vi "Test.vi"() -> ()   [LabVIEW 2014]
doc: "This VI is called when test mode begins, and will automatically be terminated when it ends. You can add manual or automatic tests and invoke them from the dashboard."
uses:
  SensorTestData.ctl
  <vilib>/Rock Robotics/WPI/Ultrasonic/WPI_SonarMB1010DigitalRefNum Registry Get.vi
  <vilib>/Rock Robotics/WPI/Ultrasonic/WPI_SonarMB1010DigitalGetRange.vi
  GyroGlobal.vi
  Elevator System/Public/Sensors Global.vi
  <vilib>/Rock Robotics/Network Tables/SD Write String.vi
  <vilib>/Rock Robotics/WPI/Joystick/WPI_JoystickGetSetRefNum.vi
  <vilib>/Rock Robotics/Network Tables/SD Write Number.vi
  <vilib>/Rock Robotics/WPI/RobotDrive/WPI_RobotDriveGetSetRefNum.vi
  <vilib>/Rock Robotics/Network Tables/SD Write Numeric Array.vi
panel:
  in  "Gripper Power":dbl=0.5 format="%#_13g"
  in  "Elevator Power":dbl=0.5 format="%#_13g"
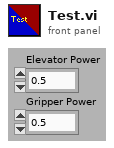
[diagram p1: front panel]
types:
  T1 = typedef "SensorTestData.ctl" = cluster{"EncoderR":dbl, "EncoderL":dbl, "EncoderS":dbl, "Tote Position":bool, "UltrasonicLR":dbl, "UltrasonicHR":dbl, "Gyro Angle":dbl, "Elevator Sensor":dbl, "Gripper Sensor L":dbl, "Gripper Sensor R":dbl}
  T2 = typedef "WPI_PotentiometerDevRef.ctl" = cluster{"DevStatus":errorcluster, "Controller":T3, "Analog Channel":T4, "Invert Output":bool}
  T3 = typedef "FPGA_TypedefAnalogModule.ctl" = enum16{"Controller 1"}
  T4 = typedef "FPGA_AIChannel.ctl" = enum8{"AI 0", "AI 1", "AI 2", "AI 3", "AI MXP 0", "AI MXP 1", "AI MXP 2", "AI MXP 3", "Invalid"}
  T5 = typedef "WPI_EncoderDevRef.ctl" = cluster{"DevStatus":errorcluster, "EncoderIndex":T6, "CounterIndex":T7, "DistancePerCount":dbl, "Decoding Type":T8}
  T6 = typedef "FPGA_EncoderIdx.ctl" = enum8{"Enc 0", "Enc 1", "Enc 2", "Enc 3", "Enc 4", "Enc 5", "Enc 6", "Enc 7", "Invalid"}
  T7 = typedef "FPGA_CounterCtrSystemIndex.ctl" = enum8{"Ctr 0", "Ctr 1", "Ctr 2", "Ctr 3", "Ctr 4", "Ctr 5", "Ctr 6", "Ctr 7", "Invalid"}
  T8 = typedef "WPI_EncoderType.ctl" = enum16{"1x", "2x", "4x"}
  T9 = typedef "WPI_SwitchDevRef.ctl" = cluster{"DevStatus":errorcluster, "DIO Channel":T10, "Controller":T11, "CntIndex":T7, "Normally Closed":bool}
  T10 = typedef "FPGA_DIOChannel.ctl" = enum8{"DIO 0", "DIO 1", "DIO 2", "DIO 3", "DIO 4", "DIO 5", "DIO 6", "DIO 7", "DIO 8", "DIO 9", "DIO MXP 0", "DIO MXP 1", "DIO MXP 2", "DIO MXP 3", "DIO MXP 4", "DIO MXP 5", "DIO MXP 6", "DIO MXP 7", "DIO MXP 8", "DIO MXP 9", "DIO MXP 10", "DIO MXP 11", "DIO MXP 12", "DIO MXP 13", "DIO MXP 14", "DIO MXP 15", "Invalid"}
  T11 = typedef "FPGA_TypedefDigitalModule.ctl" = enum16{"Controller 1"}
  T12 = typedef "WPI_SonarMB1010DigitalDeviceRef.ctl" = cluster{"CounterDevRef":T13, "Scaling factor (s/in)":dbl}
  T13 = typedef "WPI_CounterDevRef.ctl" = cluster{"DevStatus":errorcluster, "CntIndex":T7}
  T14 = typedef "WPI_JoystickDevRef.ctl" = cluster{"Device":T15}
  T15 = typedef "WPI_JoystickDeviceEnum.ctl" = enum16{"USB 0", "USB 1", "USB 2", "USB 3", "USB 4", "USB 5"}
  T16 = typedef "WPI_RobotDriveDevRef.ctl" = cluster{"DevStatus":errorcluster, "Motors[]":T17[], "Square Inputs":bool, "Max Output":dbl}
  T17 = typedef "WPI_MotorControlDeviceRef.ctl" = cluster{"DeviceStatus":errorcluster, "Type":T18, "PWM":cluster{"Controller":T11, "PWM Channel":T19, "DeadBand":T20}, "CAN":cluster{"Device Number":u8, "Control Mode":T21, "Semaphore":T22, "Max Vout":dbl, "TalonSRX Control Mode":T23}, "Invert":bool, "TransformRef":T24, "InvTransformRef":T24}
  T18 = typedef "WPI_MotorControlType.ctl" = enum16{"PWM", "CAN", "CANTalonSRX"}
  T19 = typedef "FPGA_DIOPWMChannel.ctl" = enum8{"PWM 0", "PWM 1", "PWM 2", "PWM 3", "PWM 4", "PWM 5", "PWM 6", "PWM 7", "PWM 8", "PWM 9", "PWM MXP 0", "PWM MXP 1", "PWM MXP 2", "PWM MXP 3", "PWM MXP 4", "PWM MXP 5", "PWM MXP 6", "PWM MXP 7", "PWM MXP 8", "PWM MXP 9", "Invalid"}
  T20 = typedef "WPI_PWMDeadband.ctl" = cluster{"Name":string, "maxPositivePwm":i32, "minPositivePwm":i32, "centerPwm":i32, "maxNegativePwm":i32, "minNegativePwm":i32, "angularRange":u16}
  T21 = typedef "WPI_CANJaguar_ControlMode.ctl" = enum8{"Percent VBus", "Current", "Speed", "Position", "Voltage"}
  T22 = typedef "Semaphore RefNum" = refnum<k1>
  T23 = typedef "WPI_CANTalonSRX_APIControlMode.ctl" = enum8{"Percent VBus", "Speed", "Position", "Slave", "Unchanged / Invalid"}
  T24 = typedef "WPI_PWMTransform_ConPane.ctl" = refnum<vi>
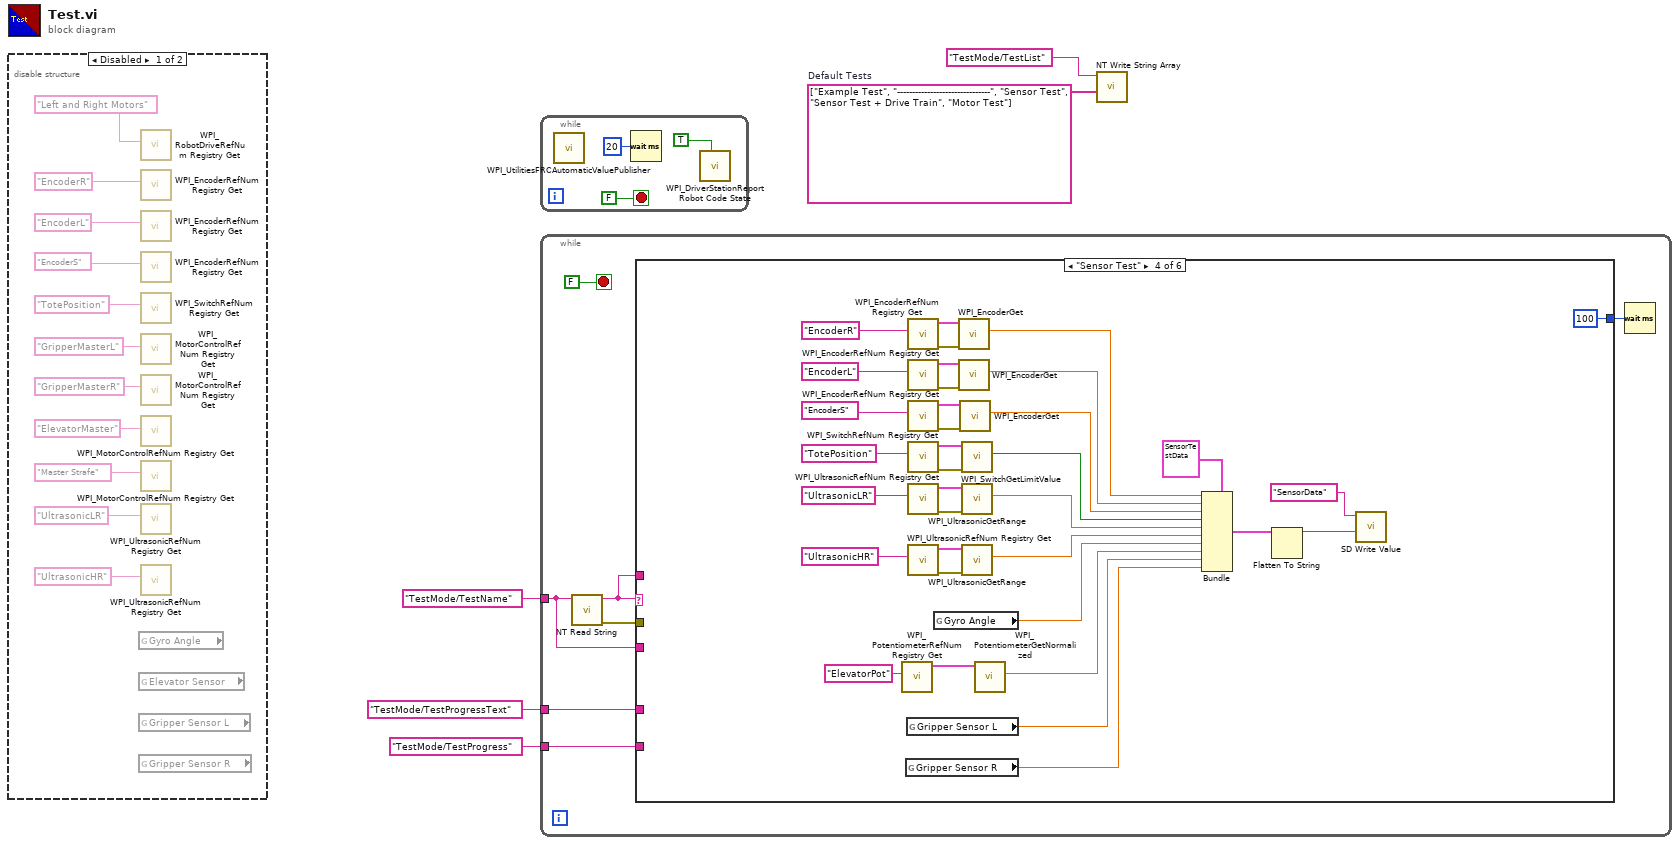
[diagram p0: block diagram]
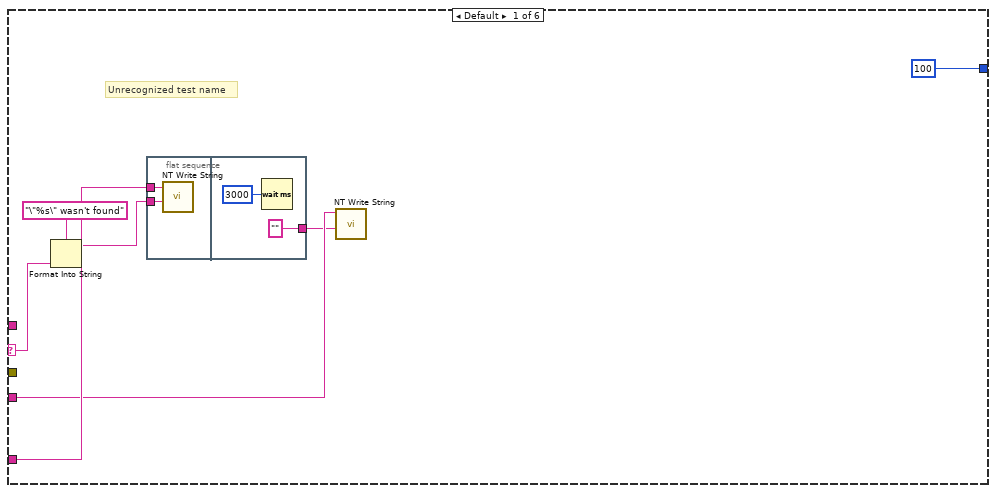
[diagram p3: hidden frame]
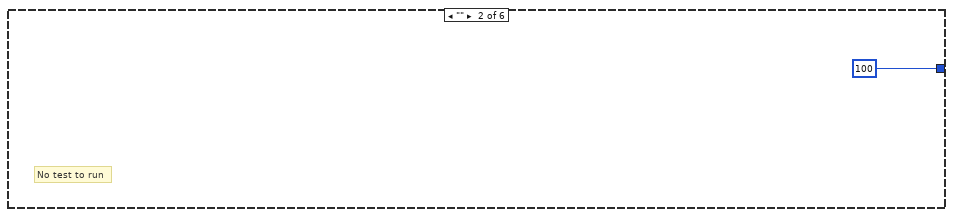
[diagram p4: hidden frame]
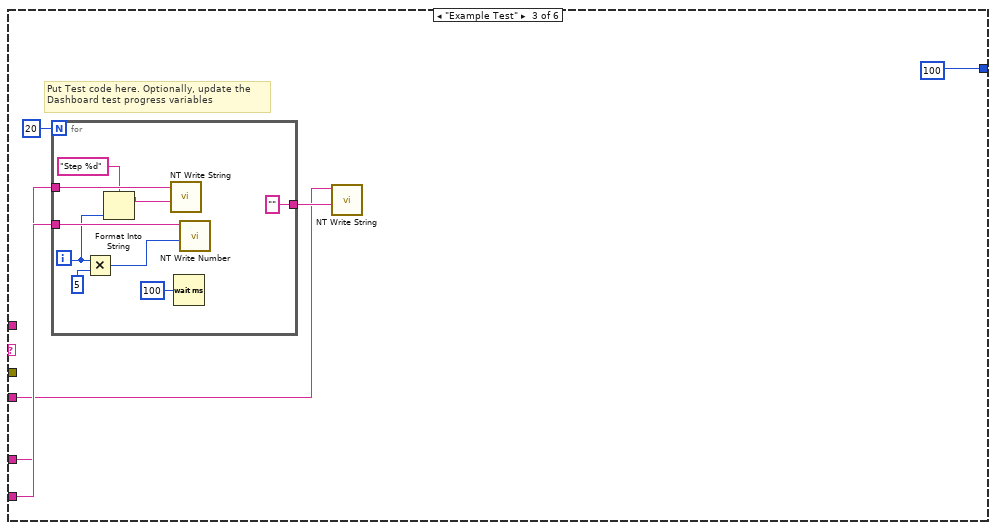
[diagram p5: hidden frame]
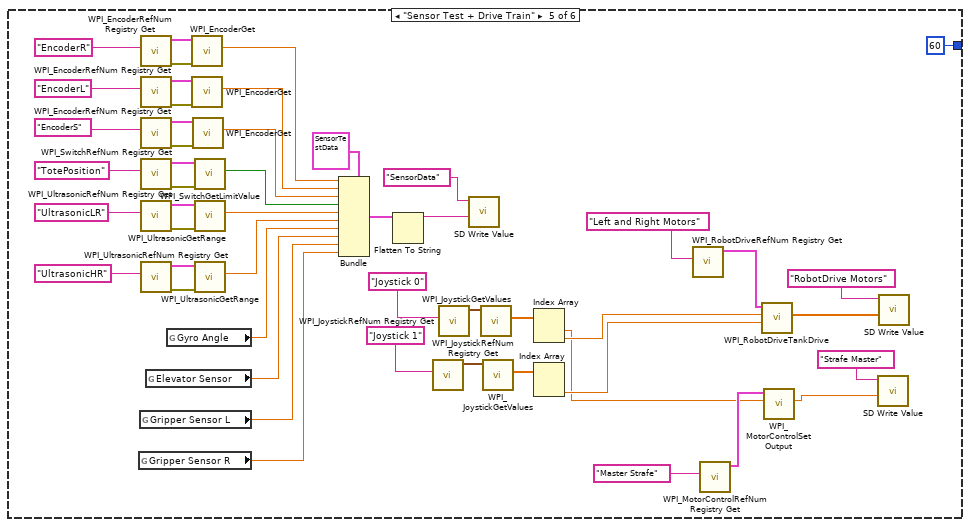
[diagram p6: hidden frame]
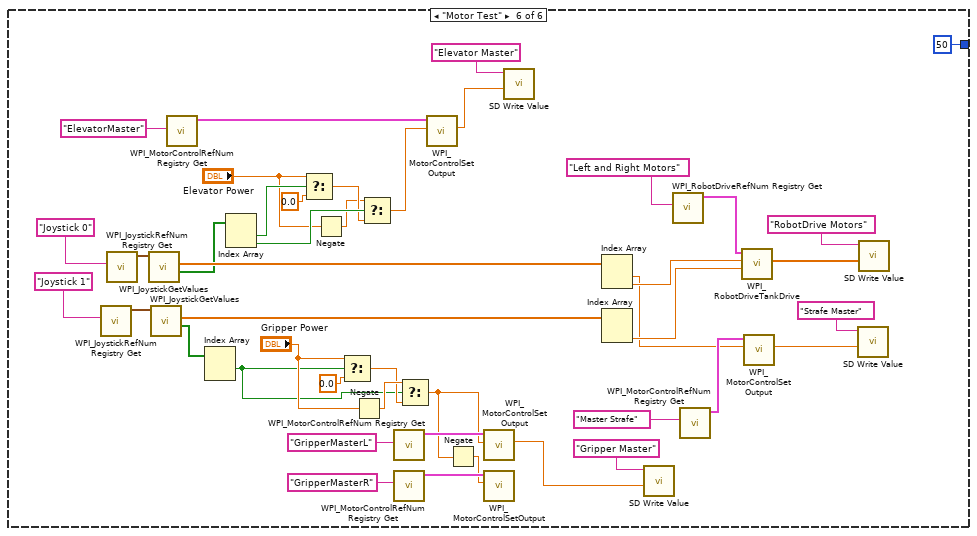
[diagram p7: hidden frame]
diagram:
  w2 = string[] ["Example Test", "-------------------------------", "Sensor Test", "Sensor Test + Drive Train", "Motor Test"]  # Default Tests
  n1 = disable-structure shown="Disabled" {
    frame Disabled {
      n2 = global read "GyroGlobal.vi" "Gyro Angle"() -> ()  [unwired: 1 out]
      n3 = global read "Sensors Global.vi" "Elevator Sensor"() -> ()  [unwired: 1 out]
      n4 = global read "Sensors Global.vi" "Gripper Sensor L"() -> ()  [unwired: 1 out]
      n5 = global read "Sensors Global.vi" "Gripper Sensor R"() -> ()  [unwired: 1 out]
      n6 = call <vilib>:"WPI_RobotDriveRefNum Registry Get.vi"("refnum name"="Left and Right Motors") -> ()  [unwired: 9 in, 2 out]
      n7 = call <vilib>:"WPI_EncoderRefNum Registry Get.vi"("refnum name"="EncoderR") -> ()  [unwired: 9 in, 2 out]
      n8 = call <vilib>:"WPI_EncoderRefNum Registry Get.vi"("refnum name"="EncoderL") -> ()  [unwired: 9 in, 2 out]
      n9 = call <vilib>:"WPI_EncoderRefNum Registry Get.vi"("refnum name"="EncoderS") -> ()  [unwired: 9 in, 2 out]
      n10 = call <vilib>:"WPI_SwitchRefNum Registry Get.vi"("refnum name"="TotePosition") -> ()  [unwired: 9 in, 2 out]
      n11 = call <vilib>:"WPI_MotorControlRefNum Registry Get.vi"("refnum name"="GripperMasterL") -> ()  [unwired: 9 in, 2 out]
      n12 = call <vilib>:"WPI_MotorControlRefNum Registry Get.vi"("refnum name"="GripperMasterR") -> ()  [unwired: 9 in, 2 out]
      n13 = call <vilib>:"WPI_MotorControlRefNum Registry Get.vi"("refnum name"="ElevatorMaster") -> ()  [unwired: 9 in, 2 out]
      n14 = call <vilib>:"WPI_MotorControlRefNum Registry Get.vi"("refnum name"="Master Strafe") -> ()  [unwired: 9 in, 2 out]
      n15 = call-poly <vilib>:"WPI_UltrasonicRefNum Registry Get.vi"("refnum name"="UltrasonicLR") -> ()  [unwired: 9 in, 2 out]
      n16 = call-poly <vilib>:"WPI_UltrasonicRefNum Registry Get.vi"("refnum name"="UltrasonicHR") -> ()  [unwired: 9 in, 2 out]
    }
    frame Enabled {
    }
  }
  n17 = while {
    stop <- FALSE stop-if-true
    n18 = call <vilib>:"WPI_UtilitiesFRCAutomaticValuePublisher.vi"() -> ()  [unwired: 12 in]
    n19 = Wait (ms)(milliseconds to wait=u32 20) -> ()  [unwired: 1 out]
    n20 = call <vilib>:"WPI_DriverStationReport Robot Code State.vi"("Test"=TRUE ("Autonomous")) -> ()  [unwired: 10 in, 1 out]
  }
  n21 = while {
    tunnel: "TestMode/TestName" ("Name") -> [w22]
    tunnel: "TestMode/TestProgressText" ("Name") -> [w25]
    tunnel: "TestMode/TestProgress" ("Name") -> [w24]
    stop <- FALSE stop-if-true
    n22 = call <vilib>:"NT Read String.vi"("Name"=w22) -> ("error out"=w21:errorcluster, "String"=w23:string)  [unwired: 9 in]
    n23 = case shown="\"Sensor Test\"" w23 {
      selector: w23 -> [w32 _ _ _ _ _]
      tunnel: w22 -> [w29 _ w40 _ _ _]
      tunnel: w25 -> [w33 _ w43 _ _ _]
      tunnel: w24 -> [_ _ w44 _ _ _]
      tunnel: w23 -> [_ _ _ _ _ _]
      tunnel: w21 -> [_ _ _ _ _ _]
      tunnel: [u32 100 ("milliseconds to wait") u32 100 ("milliseconds to wait") u32 100 ("milliseconds to wait") u32 100 ("milliseconds to wait") u32 60 ("milliseconds to wait") u32 50 ("milliseconds to wait")] -> w20
      frame Default {
        # "Unrecognized test name"
        n24 = Format Into String(format string="\"%s\" wasn't found" ("Name"), w32) -> (resulting string=w31:string)  [unwired: 2 in, 1 out]
        n25 = flat-sequence {
          tunnel: w33 -> [w34]
          tunnel: w31 -> [w35]
          tunnel: ["" ("Name")] -> w28
          frame #0 {
            n26 = call <vilib>:"NT Write String.vi"("String"=w35, "Name"=w34) -> ()  [unwired: 9 in, 1 out]
          }
          frame #1 {
            n27 = Wait (ms)(milliseconds to wait=u32 3000) -> ()  [unwired: 1 out]
          }
        }
        n28 = call <vilib>:"NT Write String.vi"("String"=w28, "Name"=w29) -> ()  [unwired: 9 in, 1 out]
      }
      frame "" {
        # "No test to run"
      }
      frame "Example Test" {
        # "Put Test code here. Optionally, update the\nDashboard test progress variables"
        n29 = for {
          N: 20 -> [_]
          tunnel: w44 -> [w53]
          tunnel: w43 -> [w51]
          tunnel: ["" ("String")] -> w41
          i -> [w48]
          n30 = Multiply(x=w48, y=u32 5 ("milliseconds to wait")) -> (x*y=w49:u32)
          n31 = Format Into String(format string="Step %d", w48) -> (resulting string=w46:string)  [unwired: 2 in, 1 out]
          n32 = call <vilib>:"NT Write String.vi"("String"=w46, "Name"=w51) -> ()  [unwired: 9 in, 1 out]
          n33 = Wait (ms)(milliseconds to wait=u32 100) -> ()  [unwired: 1 out]
          n34 = call <vilib>:"NT Write Number.vi"("Numeric"=w49, "Name"=w53) -> ()  [unwired: 9 in, 1 out]
        }
        n35 = call <vilib>:"NT Write String.vi"("String"=w41, "Name"=w40) -> ()  [unwired: 9 in, 1 out]
      }
      frame "Sensor Test" {
        n36 = call <vilib>:"WPI_PotentiometerRefNum Registry Get.vi"("refnum name"="ElevatorPot") -> ("PotDevRef"=w55:T2)  [unwired: 9 in, 1 out]
        n37 = global read "Sensors Global.vi" "Gripper Sensor R"() -> (w61:dbl)
        n38 = global read "Sensors Global.vi" "Gripper Sensor L"() -> (w62:dbl)
        n39 = call <vilib>:"WPI_EncoderRefNum Registry Get.vi"("refnum name"="EncoderR") -> ("error out"=w81:errorcluster, "EncoderDevRef"=w80:T5)  [unwired: 9 in]
        n40 = call <vilib>:"WPI_EncoderRefNum Registry Get.vi"("refnum name"="EncoderL") -> ("error out"=w79:errorcluster, "EncoderDevRef"=w78:T5)  [unwired: 9 in]
        n41 = call <vilib>:"WPI_EncoderRefNum Registry Get.vi"("refnum name"="EncoderS") -> ("error out"=w77:errorcluster, "EncoderDevRef"=w76:T5)  [unwired: 9 in]
        n42 = call <vilib>:"WPI_SwitchRefNum Registry Get.vi"("refnum name"="TotePosition") -> ("error out"=w75:errorcluster, "SwitchDevRef"=w74:T9)  [unwired: 9 in]
        n43 = call-poly <vilib>:"WPI_UltrasonicRefNum Registry Get.vi"("refnum name"="UltrasonicLR") -> ("error out"=w73:errorcluster, "SonarMB1010DigitalDevRef"=w72:T12)  [unwired: 9 in]
        n44 = call-poly <vilib>:"WPI_UltrasonicRefNum Registry Get.vi"("refnum name"="UltrasonicHR") -> ("error out"=w71:errorcluster, "SonarMB1010DigitalDevRef"=w70:T12)  [unwired: 9 in]
        n45 = global read "GyroGlobal.vi" "Gyro Angle"() -> (w63:dbl)
        n46 = call <vilib>:"WPI_EncoderGet.vi"("error in (no error)"=w81, "EncoderDevRef"=w80) -> ("Distance"=w69:dbl)  [unwired: 4 in, 5 out]
        n47 = call <vilib>:"WPI_EncoderGet.vi"("error in (no error)"=w79, "EncoderDevRef"=w78) -> ("Distance"=w68:dbl)  [unwired: 4 in, 5 out]
        n48 = call <vilib>:"WPI_EncoderGet.vi"("error in (no error)"=w77, "EncoderDevRef"=w76) -> ("Distance"=w67:dbl)  [unwired: 4 in, 5 out]
        n49 = call <vilib>:"WPI_SwitchGetLimitValue.vi"("error in (no error)"=w75, "SwitchDevRef"=w74) -> ("Switch Pressed"=w66:bool)  [unwired: 7 in, 2 out]
        n50 = call-poly <vilib>:"WPI_UltrasonicGetRange.vi"("error in"=w73, "SonarMB1010DigitalDevRef"=w72) -> ("Distance"=w65:dbl)  [unwired: 7 in, 2 out]
        n51 = call-poly <vilib>:"WPI_UltrasonicGetRange.vi"("error in"=w71, "SonarMB1010DigitalDevRef"=w70) -> ("Distance"=w64:dbl)  [unwired: 7 in, 2 out]
        n52 = call <vilib>:"WPI_PotentiometerGetNormalized.vi"("PotDevRef"=w55) -> ("Normalized Value"=w54:dbl)  [unwired: 8 in, 2 out]
        n53 = Bundle(cluster=T1 {"EncoderR"=0.0, "EncoderL"=0.0, "EncoderS"=0.0, "Tote Position"=FALSE, "UltrasonicLR"=0.0, "UltrasonicHR"=0.0, "Gyro Angle"=0.0, "Elevator Sensor"=0.0, "Gripper Sensor L"=0.0, "Gripper Sensor R"=0.0} ("Sensor Cluster"), "EncoderR"=w69, "EncoderL"=w68, "EncoderS"=w67, "Tote Position"=w66, "UltrasonicLR"=w65, "UltrasonicHR"=w64, "Gyro Angle"=w63, "Elevator Sensor"=w54, "Gripper Sensor L"=w62, "Gripper Sensor R"=w61) -> (w59:T1)
        n54 = Flatten To String(anything=w59) -> (data string=w58:string)  [unwired: 3 in, 2 out]
        n55 = call-poly <vilib>:"SD Write Value.vi"("String"=w58, "Name"="SensorData") -> ()  [unwired: 8 in, 2 out]
      }
      frame "Sensor Test + Drive Train" {
        n56 = global read "Sensors Global.vi" "Gripper Sensor R"() -> (w110:dbl)
        n57 = global read "Sensors Global.vi" "Gripper Sensor L"() -> (w111:dbl)
        n58 = call <vilib>:"WPI_EncoderRefNum Registry Get.vi"("refnum name"="EncoderR") -> ("error out"=w131:errorcluster, "EncoderDevRef"=w130:T5)  [unwired: 9 in]
        n59 = call <vilib>:"WPI_EncoderRefNum Registry Get.vi"("refnum name"="EncoderL") -> ("error out"=w129:errorcluster, "EncoderDevRef"=w128:T5)  [unwired: 9 in]
        n60 = call <vilib>:"WPI_EncoderRefNum Registry Get.vi"("refnum name"="EncoderS") -> ("error out"=w127:errorcluster, "EncoderDevRef"=w126:T5)  [unwired: 9 in]
        n61 = call <vilib>:"WPI_SwitchRefNum Registry Get.vi"("refnum name"="TotePosition") -> ("error out"=w125:errorcluster, "SwitchDevRef"=w124:T9)  [unwired: 9 in]
        n62 = call-poly <vilib>:"WPI_UltrasonicRefNum Registry Get.vi"("refnum name"="UltrasonicLR") -> ("error out"=w123:errorcluster, "SonarMB1010DigitalDevRef"=w122:T12)  [unwired: 9 in]
        n63 = call-poly <vilib>:"WPI_UltrasonicRefNum Registry Get.vi"("refnum name"="UltrasonicHR") -> ("error out"=w121:errorcluster, "SonarMB1010DigitalDevRef"=w120:T12)  [unwired: 9 in]
        n64 = global read "Sensors Global.vi" "Elevator Sensor"() -> (w112:dbl)
        n65 = global read "GyroGlobal.vi" "Gyro Angle"() -> (w113:dbl)
        n66 = call <vilib>:"WPI_EncoderGet.vi"("error in (no error)"=w131, "EncoderDevRef"=w130) -> ("Distance"=w119:dbl)  [unwired: 4 in, 5 out]
        n67 = call <vilib>:"WPI_EncoderGet.vi"("error in (no error)"=w129, "EncoderDevRef"=w128) -> ("Distance"=w118:dbl)  [unwired: 4 in, 5 out]
        n68 = call <vilib>:"WPI_EncoderGet.vi"("error in (no error)"=w127, "EncoderDevRef"=w126) -> ("Distance"=w117:dbl)  [unwired: 4 in, 5 out]
        n69 = call <vilib>:"WPI_SwitchGetLimitValue.vi"("error in (no error)"=w125, "SwitchDevRef"=w124) -> ("Switch Pressed"=w116:bool)  [unwired: 7 in, 2 out]
        n70 = call-poly <vilib>:"WPI_UltrasonicGetRange.vi"("error in"=w123, "SonarMB1010DigitalDevRef"=w122) -> ("Distance"=w115:dbl)  [unwired: 7 in, 2 out]
        n71 = call-poly <vilib>:"WPI_UltrasonicGetRange.vi"("error in"=w121, "SonarMB1010DigitalDevRef"=w120) -> ("Distance"=w114:dbl)  [unwired: 7 in, 2 out]
        n72 = Bundle(cluster=T1 {"EncoderR"=0.0, "EncoderL"=0.0, "EncoderS"=0.0, "Tote Position"=FALSE, "UltrasonicLR"=0.0, "UltrasonicHR"=0.0, "Gyro Angle"=0.0, "Elevator Sensor"=0.0, "Gripper Sensor L"=0.0, "Gripper Sensor R"=0.0} ("Sensor Cluster"), "EncoderR"=w119, "EncoderL"=w118, "EncoderS"=w117, "Tote Position"=w116, "UltrasonicLR"=w115, "UltrasonicHR"=w114, "Gyro Angle"=w113, "Elevator Sensor"=w112, "Gripper Sensor L"=w111, "Gripper Sensor R"=w110) -> (w108:T1)
        n73 = Flatten To String(anything=w108) -> (data string=w107:string)  [unwired: 3 in, 2 out]
        n74 = call <vilib>:"WPI_JoystickRefNum Registry Get.vi"("refnum name"="Joystick 1") -> ("JoystickDevRef"=w101:T14)  [unwired: 1 in, 9 out]
        n75 = call <vilib>:"WPI_JoystickRefNum Registry Get.vi"("refnum name"="Joystick 0") -> ("JoystickDevRef"=w102:T14)  [unwired: 1 in, 9 out]
        n76 = call-poly <vilib>:"SD Write Value.vi"("String"=w107, "Name"="SensorData") -> ()  [unwired: 8 in, 2 out]
        n77 = call <vilib>:"WPI_JoystickGetValues.vi"("JoystickDevRef"=w102) -> ("Axes"=w99:dbl[])  [unwired: 6 in, 4 out]
        n78 = call <vilib>:"WPI_JoystickGetValues.vi"("JoystickDevRef"=w101) -> ("Axes"=w98:dbl[])  [unwired: 6 in, 4 out]
        n79 = Index Array(array=w99) -> (element #1=w93:dbl, element #2=w94:dbl)  [unwired: 2 in]
        n80 = Index Array(array=w98) -> (element #2=w95:dbl)  [unwired: 2 in, 1 out]
        n81 = call <vilib>:"WPI_RobotDriveRefNum Registry Get.vi"("refnum name"="Left and Right Motors") -> ("RobotDriveDevRef"=w97:T16)  [unwired: 9 in, 1 out]
        n82 = call <vilib>:"WPI_MotorControlRefNum Registry Get.vi"("refnum name"="Master Strafe") -> ("MotorControlDevRef"=w96:T17)  [unwired: 9 in, 1 out]
        n83 = call <vilib>:"WPI_RobotDriveTankDrive.vi"("Right axis value"=w95, "Left axis value"=w94, "RobotDriveDevRef"=w97) -> ("Motor Values"=w91:dbl[])  [unwired: 6 in, 2 out]
        n84 = call <vilib>:"WPI_MotorControlSetOutput.vi"("Output"=w93, "MotorControlDevRef"=w96) -> ("Motor Output"=w89:dbl)  [unwired: 7 in, 2 out]
        n85 = call-poly <vilib>:"SD Write Value.vi"("Numeric"=w89, "Name"="Strafe Master") -> ()  [unwired: 8 in, 2 out]
        n86 = call-poly <vilib>:"SD Write Value.vi"("Numeric Array"=w91, "Name"="RobotDrive Motors") -> ()  [unwired: 8 in, 2 out]
      }
      frame "Motor Test" {
        n87 = call <vilib>:"WPI_JoystickRefNum Registry Get.vi"("refnum name"="Joystick 1") -> ("JoystickDevRef"=w178:T14)  [unwired: 1 in, 9 out]
        n88 = call <vilib>:"WPI_JoystickRefNum Registry Get.vi"("refnum name"="Joystick 0") -> ("JoystickDevRef"=w179:T14)  [unwired: 1 in, 9 out]
        n89 = call <vilib>:"WPI_JoystickGetValues.vi"("JoystickDevRef"=w179) -> ("Buttons"=w164:bool[], "Axes"=w176:dbl[])  [unwired: 6 in, 3 out]
        n90 = call <vilib>:"WPI_JoystickGetValues.vi"("JoystickDevRef"=w178) -> ("Buttons"=w165:bool[], "Axes"=w175:dbl[])  [unwired: 6 in, 3 out]
        n91 = call <vilib>:"WPI_MotorControlRefNum Registry Get.vi"("refnum name"="ElevatorMaster") -> ("MotorControlDevRef"=w152:T17)  [unwired: 9 in, 1 out]
        n92 = Index Array(array=w165) -> (element #1=w147:bool)  [unwired: 2 in, 1 out]
        n93 = Index Array(array=w164) -> (element #1=w159:bool, element #2=w158:bool)  [unwired: 2 in]
        n94 = Select(t="Elevator Power", s=w159, f=0.0) -> (s? t:f=w155:dbl)
        n95 = Negate(x="Elevator Power") -> (-x=w154:dbl)
        n96 = Select(t="Gripper Power", s=w147, f=0.0) -> (s? t:f=w150:dbl)
        n97 = Negate(x="Gripper Power") -> (-x=w151:dbl)
        n98 = Select(t=w154, s=w158, f=w155) -> (s? t:f=w153:dbl)
        n99 = call <vilib>:"WPI_MotorControlRefNum Registry Get.vi"("refnum name"="GripperMasterL") -> ("MotorControlDevRef"=w146:T17)  [unwired: 9 in, 1 out]
        n100 = call <vilib>:"WPI_MotorControlRefNum Registry Get.vi"("refnum name"="GripperMasterR") -> ("MotorControlDevRef"=w145:T17)  [unwired: 9 in, 1 out]
        n101 = Select(t=w151, s=w147, f=w150) -> (s? t:f=w144:dbl)
        n102 = call <vilib>:"WPI_MotorControlSetOutput.vi"("Output"=w153, "MotorControlDevRef"=w152) -> ("Motor Output"=w141:dbl)  [unwired: 7 in, 2 out]
        n103 = Negate(x=w144) -> (-x=w143:dbl)
        n104 = call <vilib>:"WPI_MotorControlSetOutput.vi"("Output"=w144, "MotorControlDevRef"=w146) -> ("Motor Output"=w139:dbl)  [unwired: 7 in, 2 out]
        n105 = call <vilib>:"WPI_MotorControlSetOutput.vi"("Output"=w143, "MotorControlDevRef"=w145) -> ()  [unwired: 7 in, 3 out]
        n106 = call-poly <vilib>:"SD Write Value.vi"("Numeric"=w141, "Name"="Elevator Master") -> ()  [unwired: 8 in, 2 out]
        n107 = Index Array(array=w176) -> (element #1=w170:dbl, element #2=w171:dbl)  [unwired: 2 in]
        n108 = Index Array(array=w175) -> (element #2=w172:dbl)  [unwired: 2 in, 1 out]
        n109 = call-poly <vilib>:"SD Write Value.vi"("Numeric"=w139, "Name"="Gripper Master") -> ()  [unwired: 8 in, 2 out]
        n110 = call <vilib>:"WPI_RobotDriveRefNum Registry Get.vi"("refnum name"="Left and Right Motors") -> ("RobotDriveDevRef"=w174:T16)  [unwired: 9 in, 1 out]
        n111 = call <vilib>:"WPI_MotorControlRefNum Registry Get.vi"("refnum name"="Master Strafe") -> ("MotorControlDevRef"=w173:T17)  [unwired: 9 in, 1 out]
        n112 = call <vilib>:"WPI_RobotDriveTankDrive.vi"("Right axis value"=w172, "Left axis value"=w171, "RobotDriveDevRef"=w174) -> ("Motor Values"=w168:dbl[])  [unwired: 6 in, 2 out]
        n113 = call <vilib>:"WPI_MotorControlSetOutput.vi"("Output"=w170, "MotorControlDevRef"=w173) -> ("Motor Output"=w166:dbl)  [unwired: 7 in, 2 out]
        n114 = call-poly <vilib>:"SD Write Value.vi"("Numeric"=w166, "Name"="Strafe Master") -> ()  [unwired: 8 in, 2 out]
        n115 = call-poly <vilib>:"SD Write Value.vi"("Numeric Array"=w168, "Name"="RobotDrive Motors") -> ()  [unwired: 8 in, 2 out]
      }
    }
    n116 = Wait (ms)(milliseconds to wait=w20) -> ()  [unwired: 1 out]
  }
  n117 = call <vilib>:"NT Write String Array.vi"("String Array"=w2, "Name"="TestMode/TestList") -> ()  [unwired: 9 in, 1 out]
